vi "Parse Comments and Commands.vi"(8 "error in":errorcluster, 10 "Igor Comments and Commands":string) -> (0 "error out":errorcluster, 1 "Commands":string, 2 "Comments":string)   [LabVIEW 2016, in "LVtoITX.lvclass"]
uses:
  LVtoITX.lvclass
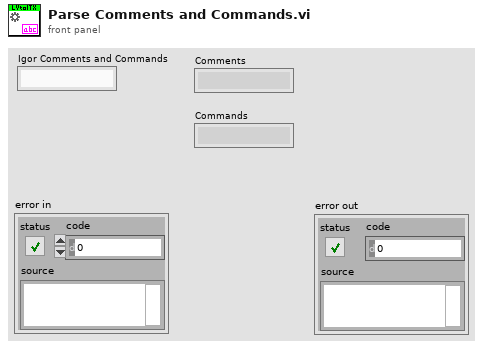
[diagram p1: front panel]
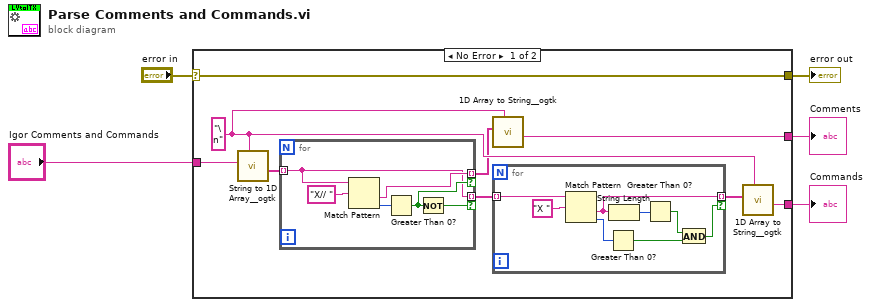
[diagram p0: block diagram]
diagram:
  n1 = case shown="No Error" "error in" {
    selector: "error in" -> [w7 w29]
    tunnel: "Igor Comments and Commands" -> [w14 _]
    tunnel: [w11 _] -> w4
    tunnel: [w7 w29] -> w2
    tunnel: [w6 _] -> w1
    frame No Error {
      w13 = "\n" ("delimiter (Tab)")
      n2 = call <userlib>:"String to 1D Array__ogtk.vi"("delimiter (Tab)"=w13, "string"=w14) -> ("Array of Strings"=w8:string[])  [unwired: 9 in]
      n3 = for {
        tunnel: w8 -> [w23] mode=indexing
        tunnel: [w26] -> w10 mode=indexing if=w24
        tunnel: [w23] -> w9 mode=indexing if=w28
        n4 = Match Pattern(string=w23, regular expression="X// " ("String")) -> (after substring=w26:string, offset past match=w25:i32)  [unwired: 3 out]
        n5 = Greater Than 0?(x=w25) -> (x > 0?=w24:bool)
        n6 = Not(x=w24) -> (.not. x?=w28:bool)
      }
      n7 = call <userlib>:"1D Array to String__ogtk.vi"("delimiter (Tab)"=w13, "Array of Strings"=w10) -> ("delimited string"=w6:string)  [unwired: 9 in]
      n8 = for {
        tunnel: w9 -> [w21] mode=indexing
        tunnel: [w19] -> w12 mode=indexing if=w15
        n9 = Match Pattern(string=w21, regular expression="X " ("String")) -> (after substring=w19:string, offset past match=w20:i32)  [unwired: 3 out]
        n10 = Greater Than 0?(x=w20) -> (x > 0?=w16:bool)
        n11 = String Length(string=w19) -> (length=w18:i32)
        n12 = Greater Than 0?(x=w18) -> (x > 0?=w17:bool)
        n13 = And(x=w17, y=w16) -> (x .and. y?=w15:bool)
      }
      n14 = call <userlib>:"1D Array to String__ogtk.vi"("delimiter (Tab)"=w13, "Array of Strings"=w12) -> ("delimited string"=w11:string)  [unwired: 9 in]
    }
    frame Error {
    }
  }
  "Commands" <- w4
  "error out" <- w2
  "Comments" <- w1
